vi "TDMS.GetChannelsForLevelTransitionAnalysis.vi"(8 "error in (no error)":errorcluster, 11 "TDMS Ref":refnum<k34>) -> (0 "error out":errorcluster, 1 "ODH Channels":string[](array[string]), 2 "OPH Channels":string[](array[string]), 3 "TDMS Ref out":refnum<k34>)   [LabVIEW 2015, in "TestStand Analysis Steps.lvlib"]
uses:
  TestStand Analysis Steps.lvlib
  Shared/Constants.vi
  Shared/Shared.lvlib
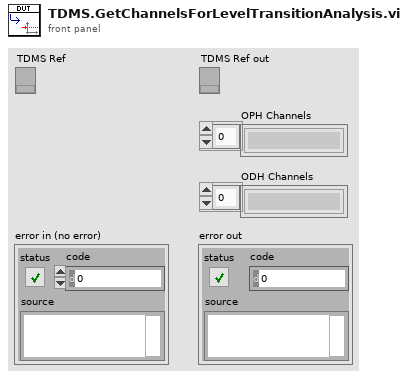
[diagram p1: front panel]
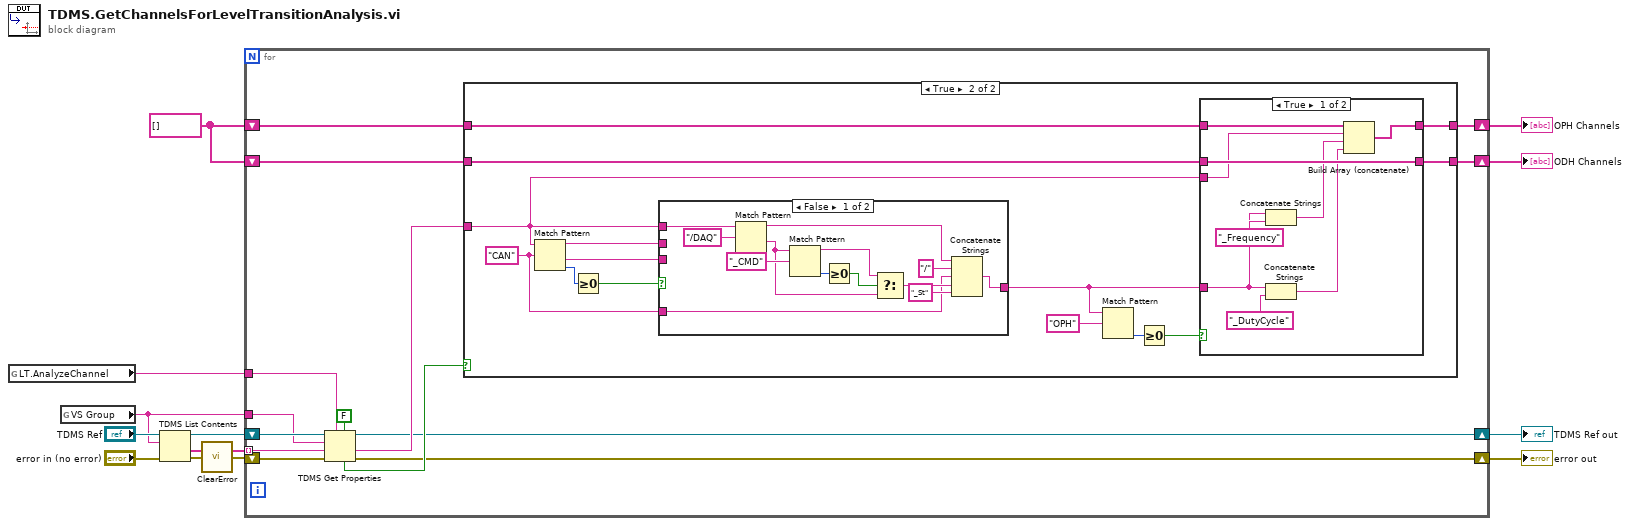
[diagram p0: block diagram]
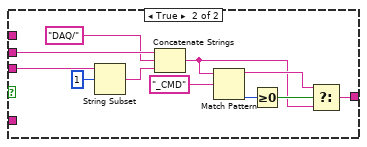
[diagram p3: hidden frame]
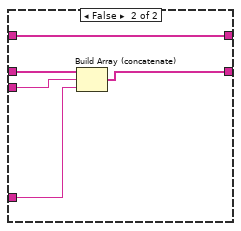
[diagram p4: hidden frame]
diagram:
  w9 = string[] []
  n1 = global read "Constants.vi" "LT.AnalyzeChannel"() -> (w1:string)
  n2 = global read "Constants.vi" "VS Group"() -> (w2:string)
  n3 = TDMS List Contents(4:"error in (no error)", 6:w2, 7:"TDMS Ref") -> (0:w3:errorcluster, 1:w8:string[], 3:w6:refnum<k34>)  [unwired: 1 out]
  n4 = call <vilib>:"ClearError.vi"("error in (no error)"=w3) -> ("error out"=w4:errorcluster)
  n5 = for {
    shift-right: [w24] -> w11
    shift-left: w9 -> [w27]
    shift-right: [w25] -> w10
    shift-left: w9 -> [w26]
    tunnel: w8 -> [w22] mode=indexing
    shift-right: [w18] -> w12
    shift-left: w6 -> [w19]
    shift-right: [w16] -> w13
    shift-left: w4 -> [w17]
    tunnel: w2 -> [w15]
    tunnel: w1 -> [w14]
    n6 = TDMS Get Properties(5:FALSE, 7:w14, 8:w17, 9:w22, 10:w15, 11:w19) -> (0:w16:errorcluster, 1:w20:string, 3:w18:refnum<k34>, 4:w21:bool)  [unwired: 2 out]
    n7 = case shown="True" w21 {
      tunnel: w20 -> [_ w30]
      tunnel: w27 -> [w29 w40]
      tunnel: w26 -> [w28 w39]
      tunnel: [w28 w38] -> w25
      tunnel: [w29 w37] -> w24
      frame False {
      }
      frame True {
        w36 = "CAN" ("regular expression")
        n8 = Match Pattern(string=w30, regular expression=w36) -> (before substring=w34:string, after substring=w35:string, offset past match=w32:i32)  [unwired: 1 in, 1 out]
        n9 = Greater Or Equal To 0?(x=w32) -> (x >= 0?=w33:bool)
        n10 = case shown="False" w33 {
          tunnel: w34 -> [_ w64]
          tunnel: w35 -> [_ w66]
          tunnel: [w53 w58] -> w31
          tunnel: w30 -> [w56 _]
          tunnel: w36 -> [w44 _]
          frame False {
            n11 = Match Pattern(string=w56, regular expression="/DAQ") -> (before substring=w45:string, after substring=w47:string)  [unwired: 1 in, 2 out]
            n12 = Match Pattern(string=w47, regular expression="_CMD") -> (before substring=w48:string, offset past match=w50:i32)  [unwired: 1 in, 2 out]
            n13 = Greater Or Equal To 0?(x=w50) -> (x >= 0?=w49:bool)
            n14 = Select(t=w48, s=w49, f=w47) -> (s? t:f=w46:string)
            n15 = Concatenate Strings(w45, "/" ("string"), w44, w46, "_St" ("string")) -> (w53:string)
          }
          frame True {
            n16 = String Subset(string=w66, offset (0)=1) -> (substring=w65:string)  [unwired: 1 in]
            n17 = Concatenate Strings(w64, "DAQ/" ("string"), w65) -> (w59:string)
            n18 = Match Pattern(string=w59, regular expression="_CMD") -> (before substring=w60:string, offset past match=w62:i32)  [unwired: 1 in, 2 out]
            n19 = Greater Or Equal To 0?(x=w62) -> (x >= 0?=w61:bool)
            n20 = Select(t=w60, s=w61, f=w59) -> (s? t:f=w58:string)
          }
        }
        n21 = Match Pattern(string=w31, regular expression="OPH") -> (offset past match=w42:i32)  [unwired: 1 in, 3 out]
        n22 = Greater Or Equal To 0?(x=w42) -> (x >= 0?=w41:bool)
        n23 = case shown="True" w41 {
          tunnel: w31 -> [w74 w80]
          tunnel: w30 -> [w71 w81]
          tunnel: w40 -> [w72 w77]
          tunnel: w39 -> [w73 w79]
          tunnel: [w73 w78] -> w38
          tunnel: [w68 w77] -> w37
          frame True {
            n24 = Concatenate Strings(w74, "_Frequency" ("string")) -> (w70:string)
            n25 = Concatenate Strings(w74, "_DutyCycle" ("string")) -> (w69:string)
            n26 = Build Array (concatenate)(w72, w71, w70, w69) -> (w68:string[])
          }
          frame False {
            n27 = Build Array (concatenate)(w79, w81, w80) -> (w78:string[])
          }
        }
      }
    }
  }
  "error out" <- w13
  "TDMS Ref out" <- w12
  "OPH Channels" <- w11
  "ODH Channels" <- w10
